vi "Close Excel sheet.vi"(5 "Completion Task":u16(ring) items=["Leave Excel Open", "Close Spreadsheet"], 7 "error out 2":errorcluster, 8 "Excel._Application":refnum<k7>, 9 "Excel._Workbook":refnum<k7>, 10 "Excel._Worksheet":refnum<k7>) -> (0 "error out":errorcluster)   [LabVIEW 2012]
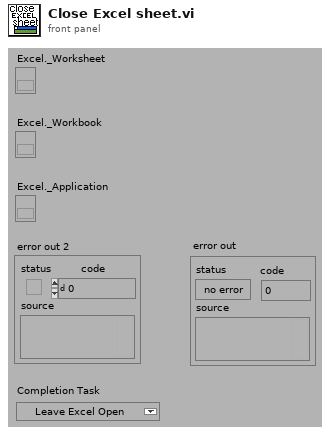
[diagram p1: front panel]
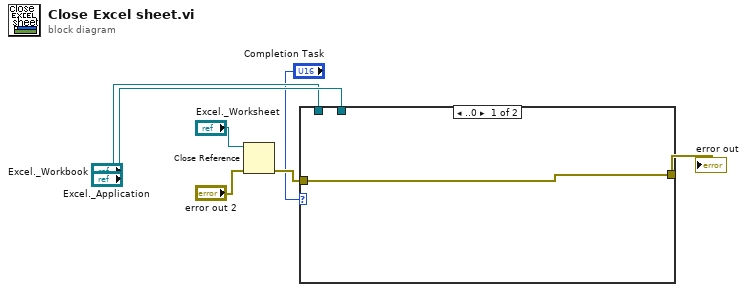
[diagram p0: block diagram]
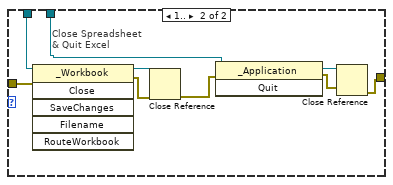
[diagram p2: hidden frame]
diagram:
  n1 = Close Reference(reference="Excel._Worksheet", error in (no error)="error out 2") -> (error out=w6:errorcluster)
  n2 = case shown="..0" "Completion Task" {
    tunnel: [w8 w9] -> w4
    tunnel: "Excel._Workbook" -> [_ w17]
    tunnel: "Excel._Application" -> [_ w13]
    tunnel: w6 -> [w8 w16]
    frame ..0 {
    }
    frame 1.. {
      # "Close Spreadsheet\n& Quit Excel"
      n3 = invoke class="_Workbook" method="Close"(reference=w17, error in=w16) -> (reference out=w15:refnum<k7>, error out=w14:errorcluster)  [unwired: 4 in, 4 out]
      n4 = Close Reference(reference=w15, error in (no error)=w14) -> (error out=w12:errorcluster)
      n5 = invoke class="_Application" method="Quit"(reference=w13, error in=w12) -> (reference out=w10:refnum<k7>, error out=w11:errorcluster)  [unwired: 1 in, 1 out]
      n6 = Close Reference(reference=w10, error in (no error)=w11) -> (error out=w9:errorcluster)
    }
  }
  "error out" <- w4
